vi "Cont Gen Voltage Wfm-Int Clk-Dig Start2.vi"() -> ()   [LabVIEW 2010]
doc: "I. Description:\nThis example demonstrates how to continuously output a waveform using an internal sample clock and a digital start trigger.\n\nII. Instructions for Running:\n1. Select the Physical Channel to correspond to where your signal is output on the DAQ device.\n2. Enter the Minimum and Maximum Voltage Ranges.\n3. Specify the Desired Frequency of the output Waveform\n4. Select the Digital Trigger Source.\n5. Specify the desired Trigger Edge.\n6. Enter the Waveform Information. See the documentation of the Waveform Buffer Generation SubVI for information on each parameter.\n\nIII. Block Diagram Steps:\n1. Create an Analog Output Voltage Task\n2.Call the DAQmx Timing (Use Waveform) VI which sets the sample clock rate based on the input waveform parameters, and set the sample mode to Continuous.\n3. Define the Triggering parameters: Source and Edge\n4. Write the waveform to the output buffer.\n5. Call the Start VI.\n6. Loop continuously until the user presses the Stop button. Check for errors every 100 ms using the Is Task Done? VI\n7. Call the Clear Task VI to clear the Task.\n8. Use the popup dialog box to display an error or warning if any.\n\nIV. I/O Connections Overview:\nMake sure your signal output terminal matches the Physical Channel I/O Control. Also, make sure your digital trigger terminal matches the Trigger Source Control. For further connection information, refer to your hardware reference manual."
uses:
  <vilib>/Utility/error.llb/DialogType.ctl
  <vilib>/DAQmx/write.llb/DAQmx Write (Analog 1D Wfm NChan NSamp).vi
  <vilib>/DAQmx/create/channels.llb/DAQmx Create Channel (AO-Voltage-Basic).vi
  <vilib>/DAQmx/configure/timing.llb/DAQmx Timing (Use Waveform).vi
  <vilib>/daqmx/miscellaneous.llb/DAQmx Fill In Error Info.vi
panel:
  out "Resulting Frequency":dbl format="%.2f"
  in  "Cycles per Buffer":i32=15
  in  "Waveform Type":T1(ring)
  in  "Amplitude":dbl=2.0 caption="Amplitude MHz" format="%0.2p"
  in  "Samples per Buffer":dbl=750.0
  in  "Desired Frequency":dbl=1000.0 format="%.2f"
  out "Output Waveform":waveform(dbl)[](graph)
  in  "Physical Channels":tag="Dev1/ao0:1"
  in  "Minimum Value":dbl=-10.0 format="%0.2f"
  in  "Maximum Value":dbl=10.0 format="%0.2f"
  in  "stop":bool
  # "For instructions, select Help>>Show Context Help"
  # "Channel Parameters"
  # "Timing Parameters"
  # "Waveform Information"
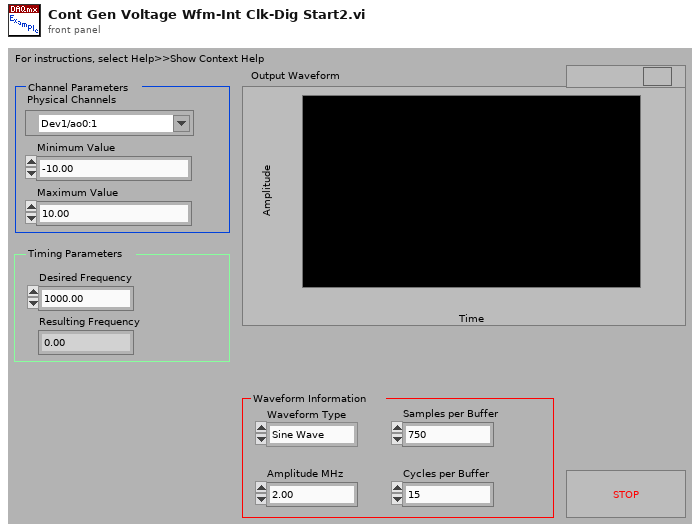
[diagram p1: front panel]
types:
  T1 = enum16{"Sine Wave", "Triangle Wave", "Square Wave", "Sawtooth Wave"}
  T2 = typedef "DialogType.ctl" = u16
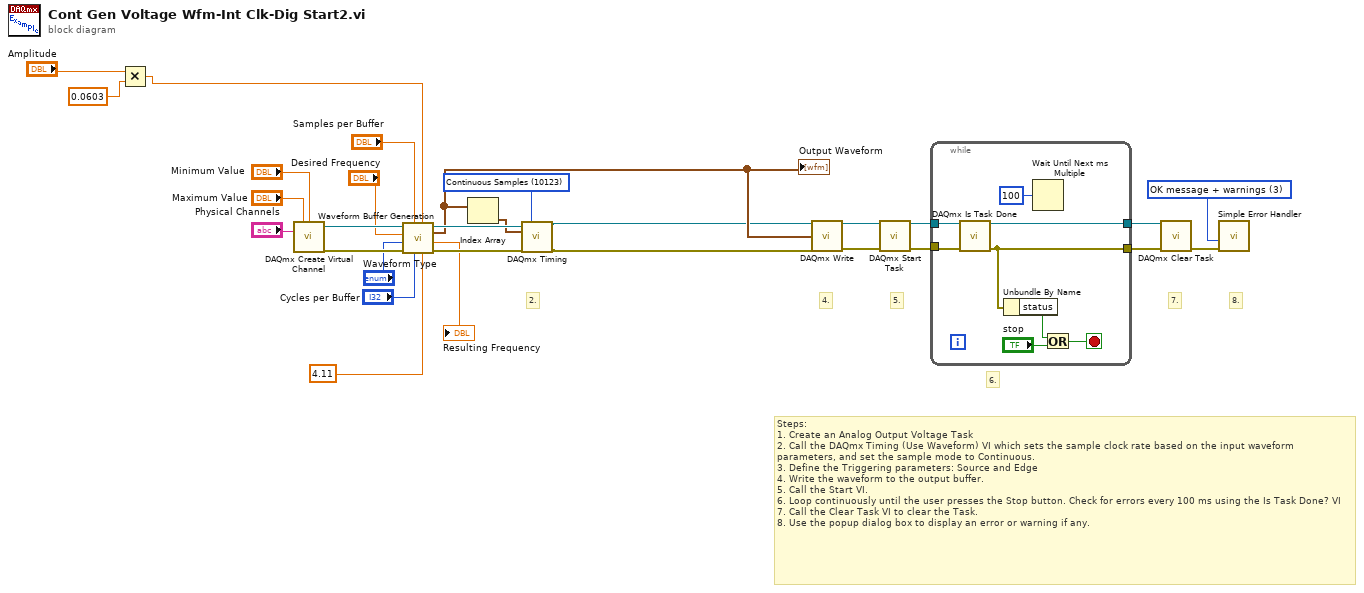
[diagram p0: block diagram]
diagram:
  w21 = T2 3 items=["no dialog", "OK message", "continue or stop message", "OK message + warnings", "continue/stop + warnings"] ("type of dialog (OK msg:1)")
  w28 = 10123 items=["Finite Samples"=10178, "Continuous Samples"=10123] ("sample mode")
  # "8."
  # "6."
  # "7."
  # "Steps: \n1. Create an Analog Output Voltage Task\n2. Call the DAQmx Timing (Use Waveform) VI which sets the sample clock rate based on the input waveform parameters, and set the sample mode to Continuous.\n3. Define the Triggering parameters: Source and Edge\n4. Write the waveform to the output buffer.\n5. Call the Start VI.\n6. Loop continuously until the user presses the Stop button. Check for errors every 100 ms using the Is Task Done? VI\n7. Call the Clear Task VI to clear the Task.\n8. Use the popup dialog box to display an error or warning if any."
  # "5."
  # "4."
  # "2."
  n1 = Multiply(x="Amplitude", y=0.0603) -> (x*y=w2:dbl)
  n2 = call-poly <vilib>:"DAQmx Create Virtual Channel.vi"("maximum value"="Maximum Value", "minimum value"="Minimum Value", "physical channels"="Physical Channels") -> ("task out"=w15:refnum<k21>, "error out"=w17:errorcluster)  [unwired: 11 in]
  n3 = call "Waveform Buffer Generation.vi"("offset"=4.11, "Amplitude"=w2, "Cycles per Buffer"="Cycles per Buffer", "Samples per Buffer"="Samples per Buffer", "error in (no error)"=w17, "Waveform Type"="Waveform Type", "Desired Frequency"="Desired Frequency", "task/channels in"=w15) -> ("error out"=w16:errorcluster, "Resulting Frequency"=→"Resulting Frequency":dbl, "Waveform"=w8:waveform(dbl)[], "task out"=w10:refnum<k21>)
  "Output Waveform" <- w8
  n4 = Index Array(array=w8) -> (element=w7:waveform(dbl))  [unwired: 1 in]
  n5 = call-poly <vilib>:"DAQmx Timing.vi"("task/channels in"=w10, "sample mode"=w28, "waveform"=w7, "error in"=w16) -> ("task out"=w6:refnum<k21>, "error out"=w5:errorcluster)  [unwired: 10 in]
  n6 = call-poly <vilib>:"DAQmx Write.vi"("task/channels in"=w6, "data"=w8, "error in"=w5) -> ("task out"=w25:refnum<k21>, "error out"=w24:errorcluster)  [unwired: 10 in, 1 out]
  n7 = call <vilib>:"DAQmx Start Task.vi"("task/channels in"=w25, "error in"=w24) -> ("task out"=w29:refnum<k21>, "error out"=w23:errorcluster)  [unwired: 12 in]
  n8 = while {
    tunnel: w29 -> [w33]
    tunnel: [w30] -> w19
    tunnel: w23 -> [w32]
    tunnel: [w31] -> w18
    stop <- w37 stop-if-true
    n9 = call <vilib>:"DAQmx Is Task Done.vi"("task/channels in"=w33, "error in"=w32) -> ("task out"=w30:refnum<k21>, "error out"=w31:errorcluster)  [unwired: 11 in, 1 out]
    n10 = Unbundle By Name(w31) -> ("status"=w35:bool)
    n11 = Wait Until Next ms Multiple(millisecond multiple=u32 100) -> ()  [unwired: 1 out]
    n12 = Or(x=w35, y="stop") -> (x .or. y?=w37:bool)
  }
  n13 = call <vilib>:"DAQmx Clear Task.vi"("task in"=w19, "error in"=w18) -> ("error out"=w20:errorcluster)  [unwired: 13 in]
  n14 = call <vilib>:"Simple Error Handler.vi"("type of dialog (OK msg:1)"=w21, "error in (no error)"=w20) -> ()  [unwired: 3 in, 5 out]
